vi "Cartesian Offsets.vi"(4 "Use Individual Lbcbs":bool, 5 "Use Offsets":bool, 9 "LBCB Number":T2) -> (1 "Cartesian Data Offsets Out":T1, 3 "Cartesian Data Out":T1)   [LabVIEW 2009]
uses:
  Global Data/Cartesian Data type.ctl
  Data Access Objects/Metadata/LBCB Number.ctl
  Global Data/Cartesian Measurment Actions.ctl
  Data Access Objects/Metadata/DAO Actions.ctl
panel:
  # "Use only when in the rigid connection configuration"
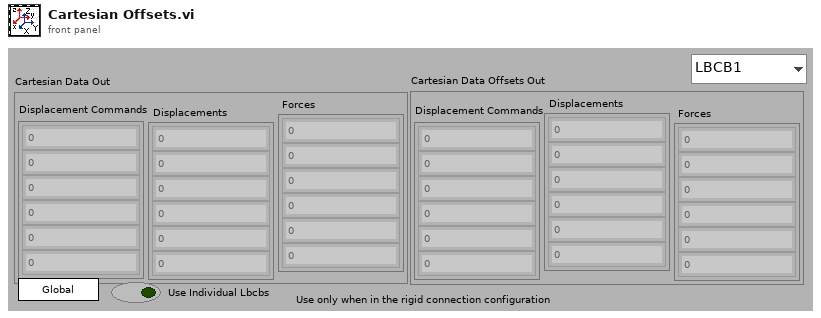
[diagram p1: front panel]
types:
  T1 = typedef "Cartesian Data Type.ctl" = cluster{"Displacements":dbl[], "Forces":dbl[], "Displacement Commands":dbl[]}
  T2 = typedef "LBCB Number.ctl" = enum16{"LBCB1", "LBCB2"}
  T3 = typedef "Cartesian Measurment Actions.ctl" = enum16{"Set Data", "Get", "Init", "Set Offsets"}
  T4 = typedef "DAO Actions.ctl" = enum16{"Init", "Get", "Set"}
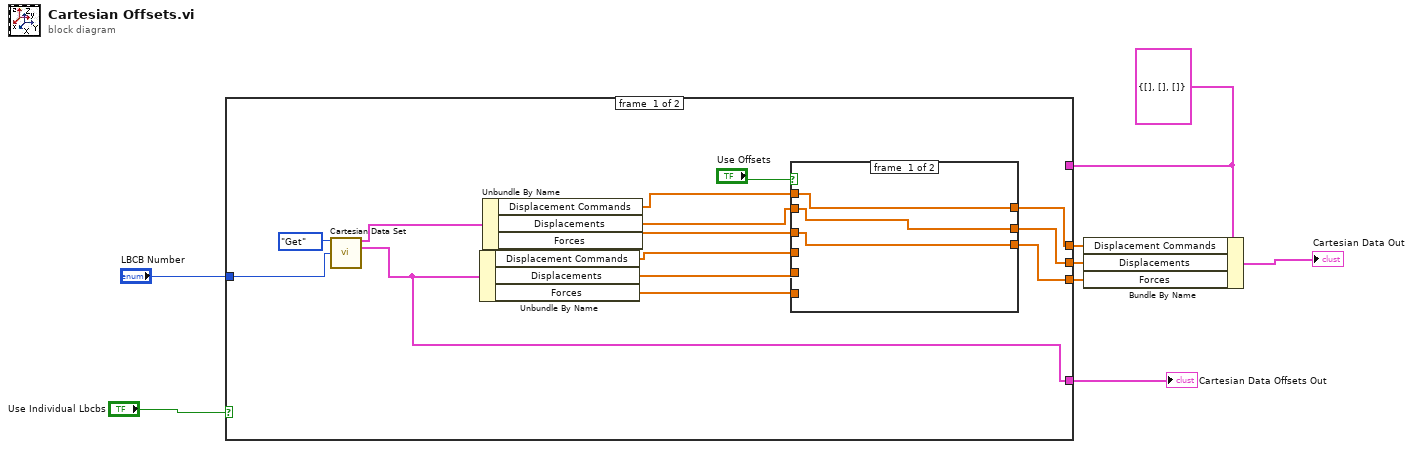
[diagram p0: block diagram]
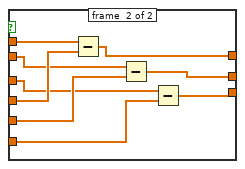
[diagram p2: hidden frame]
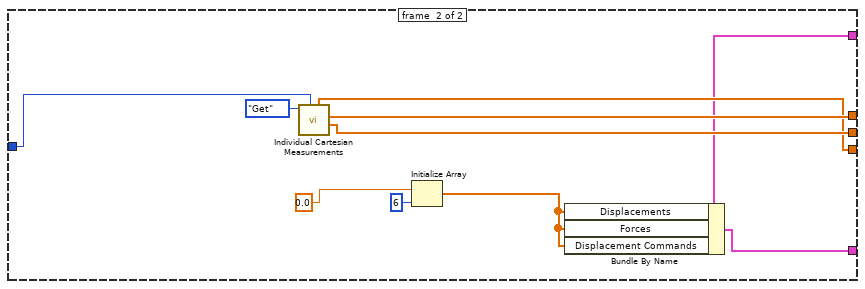
[diagram p3: hidden frame]
diagram:
  w2 = T1 {"Displacements"=[], "Forces"=[], "Displacement Commands"=[]} ("Offsets")
  n1 = case shown="False" "Use Individual Lbcbs" {
    tunnel: [w18 w41] -> w7
    tunnel: [w15 w40] -> w6
    tunnel: "LBCB Number" -> [w14 w43]
    tunnel: [w11 w42] -> w4
    tunnel: w2 -> [_ w39]
    tunnel: [w9 w35] -> w1
    frame #0 {
      n2 = call "Cartesian Data Set.vi"("Measurement Actions"=Cartesian_Measurment_Actions."Get", "LBCB Selected"=w14) -> ("Cartesian Data Out"=w10:T1, "Cartesian Data Offsets Out"=w9:T1)  [unwired: 4 in, 8 out]
      n3 = Unbundle By Name(w9) -> ("Displacement Commands"=w12:dbl[], "Displacements"=w19:dbl[], "Forces"=w16:dbl[])
      n4 = Unbundle By Name(w10) -> ("Displacement Commands"=w13:dbl[], "Displacements"=w20:dbl[], "Forces"=w17:dbl[])
      n5 = case shown="True" "Use Offsets" {
        tunnel: [w25 w34] -> w11
        tunnel: w13 -> [w25 w33]
        tunnel: w12 -> [_ w32]
        tunnel: w20 -> [w24 w31]
        tunnel: w19 -> [_ w30]
        tunnel: [w24 w29] -> w18
        tunnel: w17 -> [w23 w28]
        tunnel: w16 -> [_ w27]
        tunnel: [w23 w26] -> w15
        frame #0 {
        }
        frame #1 {
          n6 = Subtract(x=w33, y=w32) -> (x-y=w34:dbl[])
          n7 = Subtract(x=w31, y=w30) -> (x-y=w29:dbl[])
          n8 = Subtract(x=w28, y=w27) -> (x-y=w26:dbl[])
        }
      }
    }
    frame #1 {
      n9 = call "Individual Cartesian Measurements.vi"("LBCB Number"=w43, "DAO Actions"=DAO_Actions."Get") -> ("Displacements Out"=w41:dbl[], "Commands Out"=w42:dbl[], "Forces Out"=w40:dbl[])  [unwired: 6 in, 1 out]
      n10 = Initialize Array(0.0 ("Numeric"), 6 ("dimension size")) -> (w36:dbl[])
      n11 = Bundle By Name(cluster=w39, "Displacements"=w36, "Forces"=w36, "Displacement Commands"=w36) -> (w35:T1)
    }
  }
  "Cartesian Data Offsets Out" <- w1
  n12 = Bundle By Name(cluster=w2, "Displacement Commands"=w4, "Displacements"=w7, "Forces"=w6) -> (→"Cartesian Data Out":T1)
